vi "CombineSpectrumAndMedian.vi"(7 "SNR_Thresh":dbl=-90.0 caption="Don't AutoCenter below this SNR level (dB)", 10 "median":dbl, 11 "PwrSpectrum":dbl[](array[numeric])) -> (3 "Array":dbl[][](array[numeric]))   [LabVIEW 2018]
doc: "Combine Spectrum and a line at the noise median to display on a graph"
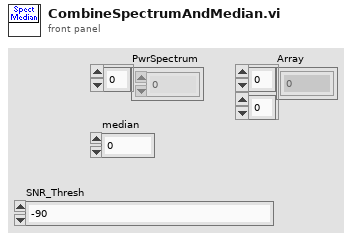
[diagram p1: front panel]
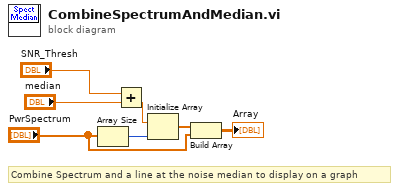
[diagram p0: block diagram]
diagram:
  # "Combine Spectrum and a line at the noise median to display on a graph"
  n1 = Array Size(array="PwrSpectrum") -> (size(s)=w4:i32)
  n2 = Add(x="SNR_Thresh", y="median") -> (x+y=w2:dbl)
  n3 = Initialize Array(w2, w4) -> (w6:dbl[])
  n4 = Build Array(w6, "PwrSpectrum") -> (→"Array":dbl[][])
